vi "Parcial1LesterRoche.vi"() -> ()   [LabVIEW 2011]
panel:
  out "promedio":dbl
  out "Mayor numero de galones":dbl
  out "701-1000":bool
  out "501-700":bool
  out "351-500":bool
  out "1-350":bool
  in  "Knob":i32(knob) scale=0.0..50.0
  out "Tanque de agua":i32(slide) scale=0.0..1000.0
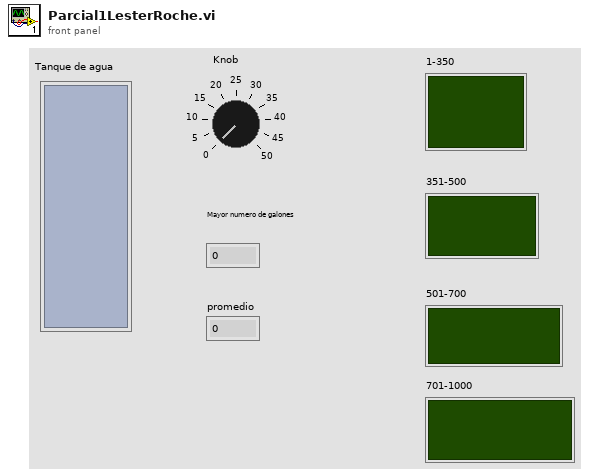
[diagram p1: front panel]
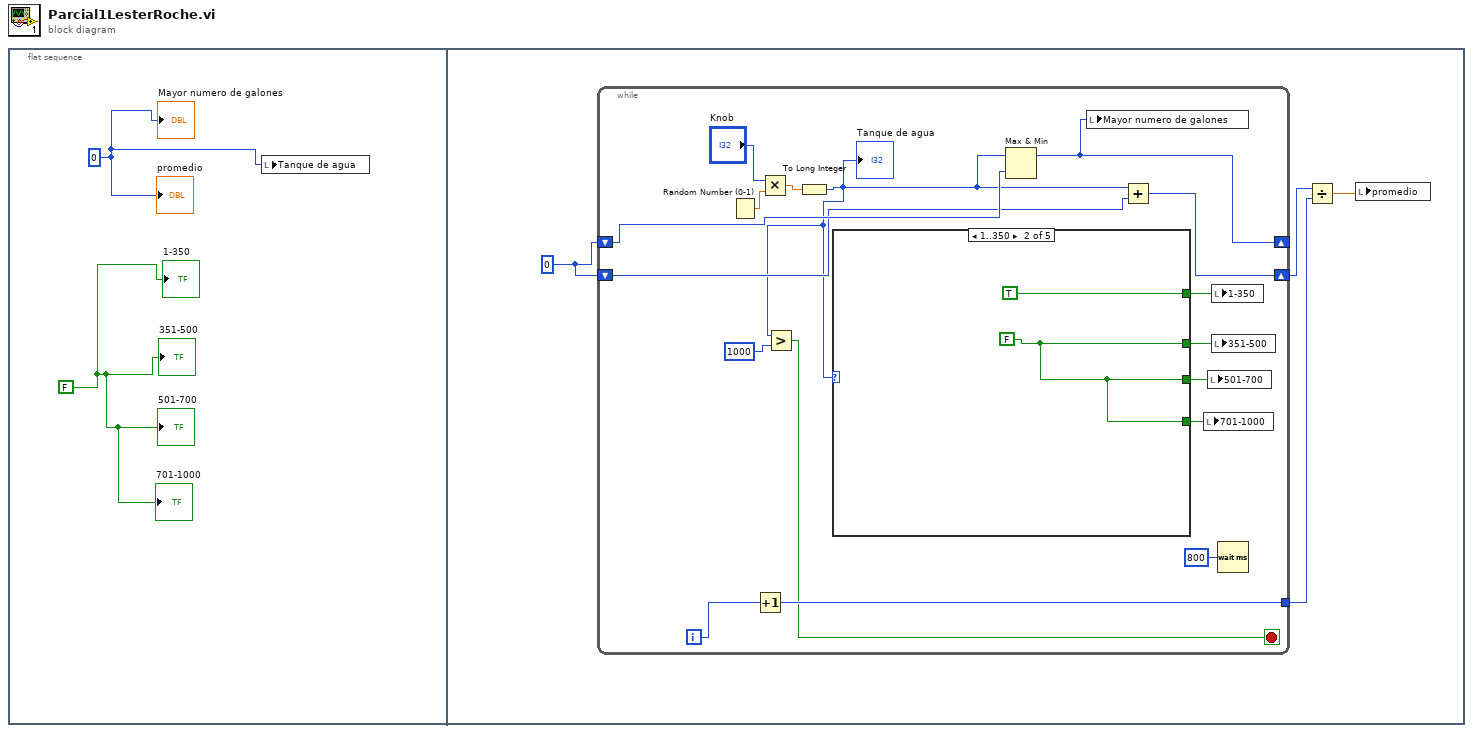
[diagram p0: block diagram]
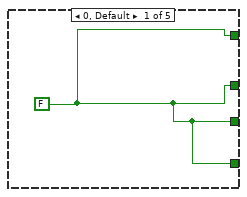
[diagram p2: hidden frame]
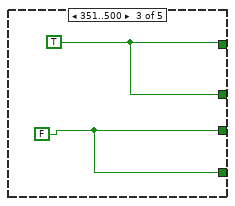
[diagram p3: hidden frame]
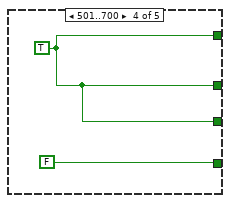
[diagram p4: hidden frame]
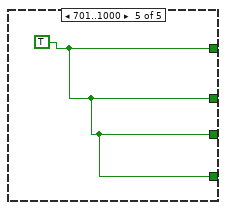
[diagram p5: hidden frame]
diagram:
  n1 = flat-sequence {
    frame #0 {
      w2 = FALSE
      w1 = 0
      n2 = local write "Tanque de agua"(w1) -> ()
      "Mayor numero de galones" <- w1
      "promedio" <- w1
      "1-350" <- w2
      "351-500" <- w2
      "501-700" <- w2
      "701-1000" <- w2
    }
    frame #1 {
      w4 = 0
      n3 = while {
        tunnel: [w14] -> w6
        shift-right: [w10] -> _
        shift-left: w4 -> [w11]
        shift-right: [w8] -> w3
        shift-left: w4 -> [w9]
        i -> [w15]
        stop <- w12 stop-if-true
        n4 = Random Number (0-1)() -> (number: 0 to 1=w22:dbl)
        n5 = Increment(x=w15) -> (x+1=w14:i32)
        n6 = Multiply(x="Knob", y=w22) -> (x*y=w21:dbl)
        n7 = To Long Integer(number=w21) -> (32bit integer=w7:i32)
        "Tanque de agua" <- w7
        n8 = Greater?(x=w7, y=1000) -> (0:w12:bool)
        n9 = case shown="1..350" w7 {
          tunnel: [w24 TRUE w28 w30 w31] -> w20
          tunnel: [w24 w25 w28 w30 w31] -> w19
          tunnel: [w24 w25 w27 w30 w31] -> w18
          tunnel: [w24 w25 w27 FALSE w31] -> w17
          frame 0, Default {
            w24 = FALSE
          }
          frame 1..350 {
            w25 = FALSE
          }
          frame 351..500 {
            w27 = FALSE
            w28 = TRUE
          }
          frame 501..700 {
            w30 = TRUE
          }
          frame 701..1000 {
            w31 = TRUE
          }
        }
        n10 = Max & Min(x=w7, y=w11) -> (max(x,y)=w10:i32)  [unwired: 1 out]
        n11 = local write "Mayor numero de galones"(w10) -> ()
        n12 = Add(x=w7, y=w9) -> (x+y=w8:i32)
        n13 = local write "701-1000"(w17) -> ()
        n14 = local write "501-700"(w18) -> ()
        n15 = local write "1-350"(w20) -> ()
        n16 = local write "351-500"(w19) -> ()
        n17 = Wait (ms)(milliseconds to wait=u32 800) -> ()  [unwired: 1 out]
      }
      n18 = Divide(x=w3, y=w6) -> (x/y=w5:dbl)
      n19 = local write "promedio"(w5) -> ()
    }
  }
